vi "AES - Get Key and IV.vi"(8 "error in (no error)":errorcluster) -> (0 "error out":errorcluster, 2 "IV":u8[](array[numeric]), 3 "Key":u8[](array[numeric]))   [LabVIEW 2013]
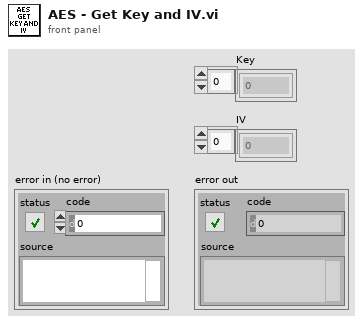
[diagram p1: front panel]
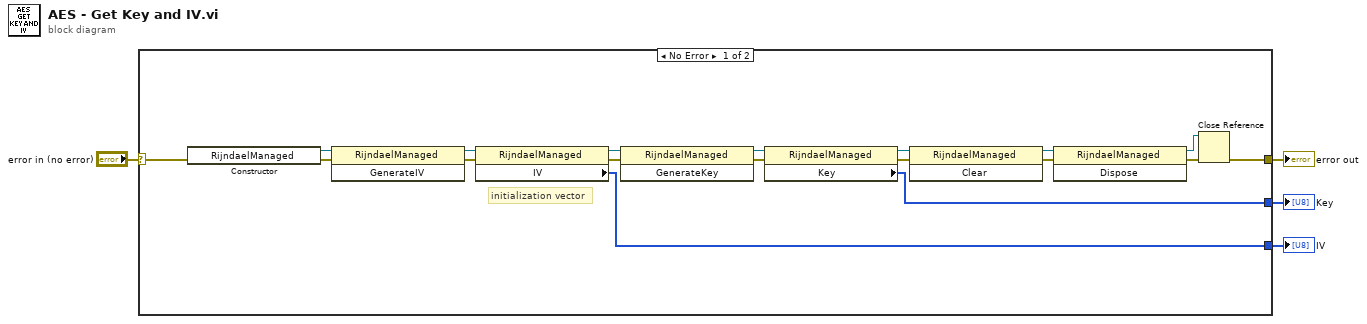
[diagram p0: block diagram]
diagram:
  n1 = case shown="No Error" "error in (no error)" {
    selector: "error in (no error)" -> [w5 w23]
    tunnel: [w8 _] -> w4
    tunnel: [w7 _] -> w3
    tunnel: [w6 w23] -> w2
    frame No Error {
      # "initialization vector"
      n2 = constructor class="RijndaelManaged"(error in=w5) -> (reference out=w22:refnum<k24>, error out=w21:errorcluster)  [unwired: 2 in, 1 out]
      n3 = invoke class="RijndaelManaged" method="GenerateIV"(reference=w22, error in=w21) -> (reference out=w20:refnum<k24>, error out=w17:errorcluster)  [unwired: 1 in, 1 out]
      n4 = property class="RijndaelManaged"(reference=w20, error in=w17) -> (reference out=w19:refnum<k24>, error out=w16:errorcluster, "IV"=w8:u8[])
      n5 = invoke class="RijndaelManaged" method="GenerateKey"(reference=w19, error in=w16) -> (reference out=w18:refnum<k24>, error out=w15:errorcluster)  [unwired: 1 in, 1 out]
      n6 = property class="RijndaelManaged"(reference=w18, error in=w15) -> (reference out=w13:refnum<k24>, error out=w12:errorcluster, "Key"=w7:u8[])
      n7 = invoke class="RijndaelManaged" method="Clear"(reference=w13, error in=w12) -> (reference out=w14:refnum<k24>, error out=w11:errorcluster)  [unwired: 1 in, 1 out]
      n8 = invoke class="RijndaelManaged" method="Dispose"(reference=w14, error in=w11) -> (reference out=w10:refnum<k24>, error out=w9:errorcluster)  [unwired: 1 in, 1 out]
      n9 = Close Reference(reference=w10, error in (no error)=w9) -> (error out=w6:errorcluster)
    }
    frame Error {
    }
  }
  "IV" <- w4
  "Key" <- w3
  "error out" <- w2
